vi "SRAD Delete 32f.vi"(8 "Error In":errorcluster, 11 "SRAD Filter Object":T1={"Device In"=0, "Program Handle"=0, "N"={"Device ID"=0, "Memeroy ID"=0, "Dimension"={"Depth"=0, "Height"=0, "Width"=0}, "Memory Type"=enum."32f"}, "N + 1"={"Device ID"=0, "Memeroy ID"=0, "Dimension"={"Depth"=0, "Height"=0, "Width"=0}, "Memory Type"=enum."32f"}, "Dimensions"={"Depth"=1, "Height"=1, "Width"=1}, "Diffusivity"={"Device ID"=0, "Memeroy ID"=0, "Dimension"={"Depth"=0, "Height"=0, "Width"=0}, "Memory Type"=enum."32f"}} {"Diffusivity"."Dimension"."Width" min=1; "Diffusivity"."Dimension"."Height" min=1; "Diffusivity"."Dimension"."Depth" min=1; "Dimensions"."Width" min=1; "Dimensions"."Height" min=1; "Dimensions"."Depth" min=1; "N + 1"."Dimension"."Width" min=1; "N + 1"."Dimension"."Height" min=1; "N + 1"."Dimension"."Depth" min=1; "N"."Dimension"."Width" min=1; "N"."Dimension"."Height" min=1; "N"."Dimension"."Depth" min=1}) -> (0 "Error Out":errorcluster)   [LabVIEW 2012, in "OpenCLV x64.lvlib"]
uses:
  OpenCLV x64.lvlib
  Controls/SRAD Filter Object.ctl
  Controls/Device ID.ctl
  Controls/Program Handle.ctl
  Controls/Memory Object.ctl
  Controls/Memory ID.ctl
  User Controls/Array Dimensions.ctl
  Controls/Memory Type.ctl
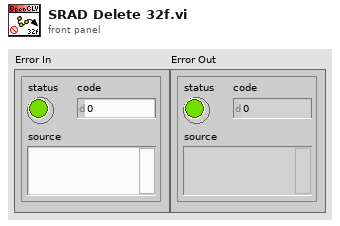
[diagram p1: front panel]
types:
  T1 = typedef "OpenCLV x64.lvlib/SRAD Filter Object.ctl" = cluster{"Device In":T2, "Program Handle":T3, "N":T4, "N + 1":T4, "Dimensions":T6, "Diffusivity":T4}
  T2 = typedef "OpenCLV x64.lvlib/Device ID.ctl" = u64
  T3 = typedef "OpenCLV x64.lvlib/Program Handle.ctl" = u64
  T4 = typedef "OpenCLV x64.lvlib/Memory Object.ctl" = cluster{"Device ID":T2, "Memeroy ID":T5, "Dimension":T6, "Memory Type":T7}
  T5 = typedef "OpenCLV x64.lvlib/Memory ID.ctl" = u64
  T6 = typedef "Array Dimensions.ctl" = cluster{"Depth":u64, "Height":u64, "Width":u64}
  T7 = typedef "OpenCLV x64.lvlib/Memory Type.ctl" = enum16{"32f", "u8", "i8", "u16", "i16", "u32", "i32", "64f"}
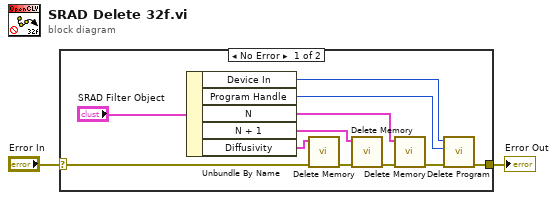
[diagram p0: block diagram]
diagram:
  n1 = case shown="No Error" "Error In" {
    selector: "Error In" -> [w4 w14]
    tunnel: [w5 w14] -> w1
    frame No Error {
      n2 = Unbundle By Name("SRAD Filter Object") -> ("Device In"=w3:T2, "Program Handle"=w7:T3, "N"=w10:T4, "N + 1"=w11:T4, "Diffusivity"=w12:T4)
      n3 = call "Delete Memory.vi"("Error In"=w4, "Memory Object In"=w12) -> ("Error Out"=w8:errorcluster)  [unwired: 8 in, 1 out]
      n4 = call "Delete Memory.vi"("Error In"=w8, "Memory Object In"=w11) -> ("Error Out"=w9:errorcluster)  [unwired: 8 in, 1 out]
      n5 = call "Delete Memory.vi"("Error In"=w9, "Memory Object In"=w10) -> ("Error Out"=w6:errorcluster)  [unwired: 8 in, 1 out]
      n6 = call "Delete Program.vi"("Error In"=w6, "Program In"=w7, "Device ID"=w3) -> ("Error Out"=w5:errorcluster)  [unwired: 8 in]
    }
    frame Error {
    }
  }
  "Error Out" <- w1
